vi "Alarm.Get.vi"(8 "error in (no error)":errorcluster, 11 "Alarm":string) -> (0 "error out":errorcluster, 3 "Alarm Data":T1 {"Trip Value" format="%.2f"; "Delay" format="%.2f"; "Low Limit" format="%.2f"; "High Limit" format="%.2f"})   [LabVIEW 2015, in "Single Station Execution.lvlib"]
uses:
  Single Station Execution.lvlib
  <vilib>/NI Veristand/Execution/Alarm/AlarmInfo.ctl
  <vilib>/NI Veristand/Execution/Alarm/NI_VS Alarm ExecutionAPI.lvlib
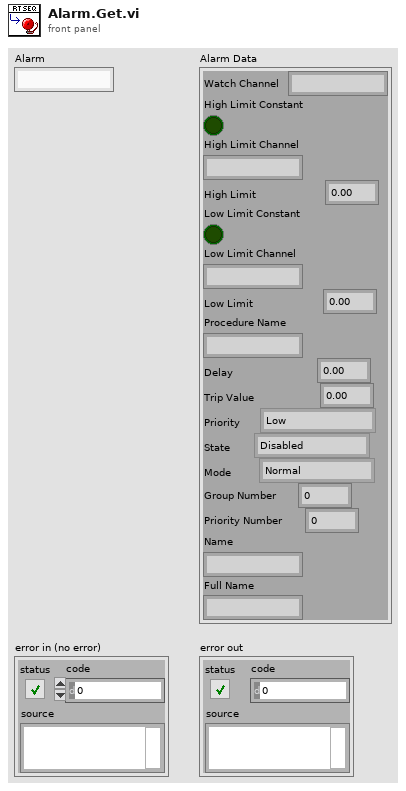
[diagram p1: front panel]
types:
  T1 = typedef "NI_VS Alarm ExecutionAPI.lvlib/AlarmInfo.ctl" = cluster{"Watch Channel":string, "High Limit Constant":bool, "High Limit Channel":string, "High Limit":dbl, "Low Limit Constant":bool, "Low Limit Channel":string, "Low Limit":dbl, "Procedure Name":string, "Delay":dbl, "Trip Value":dbl, "Priority":enum16{"Low", "Medium", "High"}, "State":enum16{"Disabled", "Enabled", "Tripped", "Delayed Trip", "Indicate"}, "Mode":enum16{"Normal", "Indicate Only"}, "Group Number":u32, "Priority Number":u32, "Name":string, "Full Name":string}
  T2 = typedef "NI_VS Alarm ExecutionAPI.lvlib/AlarmAPI.ctl" = refnum<k24>
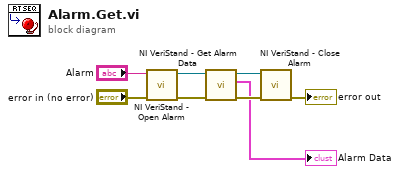
[diagram p0: block diagram]
diagram:
  n1 = call <vilib>:"NI VeriStand - Open Alarm.vi"("error in (no error)"="error in (no error)", "Alarm Name"="Alarm") -> ("error out"=w2:errorcluster, "Alarm"=w1:T2)  [unwired: 8 in]
  n2 = call <vilib>:"NI VeriStand - Get Alarm Data.vi"("error in (no error)"=w2, "Alarm in"=w1) -> ("error out"=w5:errorcluster, "Alarm Data"=→"Alarm Data":T1, "Alarm out"=w4:T2)  [unwired: 7 in]
  n3 = call <vilib>:"NI VeriStand - Close Alarm.vi"("error in (no error)"=w5, "Alarm"=w4) -> ("error out"=→"error out":errorcluster)  [unwired: 9 in]
